vi "q4 rc circuit.vi"() -> ()   [LabVIEW 2018]
panel:
  out "Waveform Chart":dynamicdata(graph)
  in  "stop (F)":bool
  in  "data":dbl
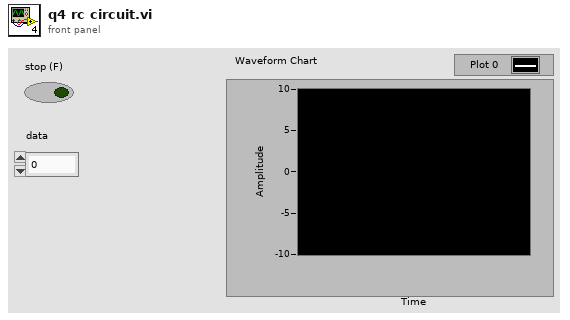
[diagram p1: front panel]
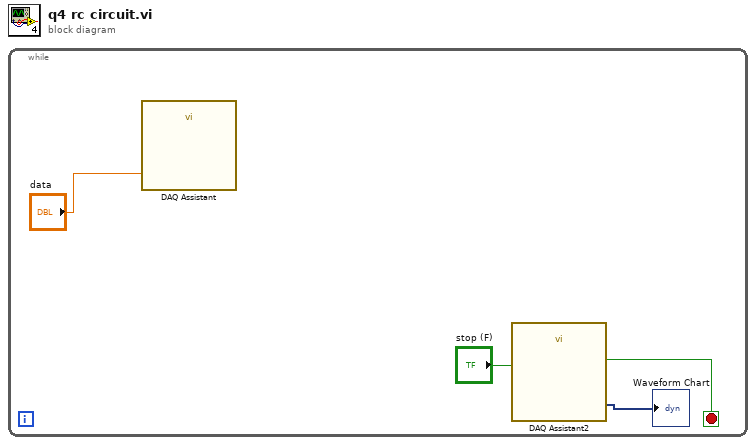
[diagram p0: block diagram]
diagram:
  n1 = while {
    stop <- w3 stop-if-true
    n2 = call "DAQ Assistant"("data"="data") -> ()  [unwired: 17 in, 2 out]
    n3 = call "DAQ Assistant2"("stop (F)"="stop (F)") -> ("data"=→"Waveform Chart":dynamicdata, "stopped"=w3:bool)  [unwired: 15 in, 2 out]
  }
